vi "regressors.calculate.vi"(6 "reset? (F)":bool, 9 "initial_value (0)":dbl, 10 "variable v(k)":dbl, 11 "b0...bn":dbl[](array[numeric])=[0.0, 0.0, 0.0, 0.0]) -> (3 "result r(k)":dbl)   [LabVIEW 2015, in "discrete_control_systems.lvlib"]
doc: "Calculates a difference equation of the form r(k) = c0*v(k) + c1*v(k-1) + c2*v(k-2) .... cn*v(k-n) \n\nThe reset? input clears registers and intializes them to the specified initial value."
uses:
  discrete_control_systems.lvlib
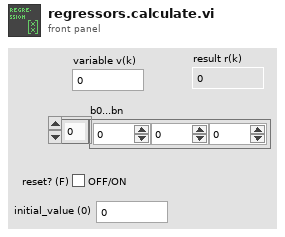
[diagram p1: front panel]
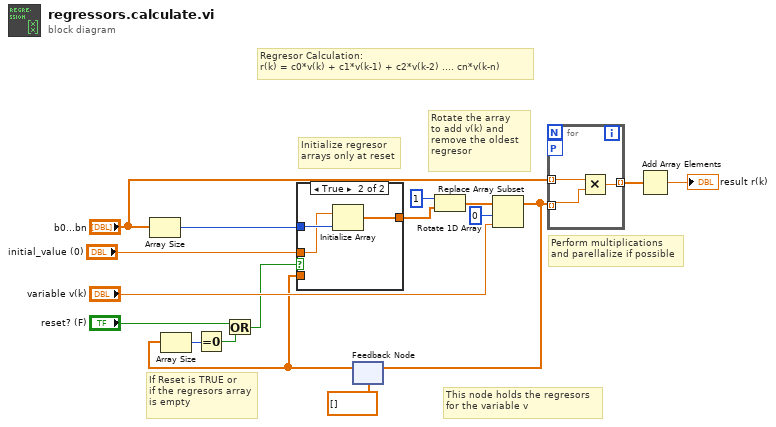
[diagram p0: block diagram]
diagram:
  # "If Reset is TRUE or\nif the regresors array\nis empty"
  # "Perform multiplications\nand parellalize if possible"
  # "Regresor Calculation:\nr(k) = c0*v(k) + c1*v(k-1) + c2*v(k-2) .... cn*v(k-n)"
  # "Initialize regresor\narrays only at reset"
  # "Rotate the array\nto add v(k) and \nremove the oldest \nregresor"
  # "This node holds the regresors\nfor the variable v"
  n1 = Array Size(array="b0...bn") -> (size(s)=w16:i32)
  n2 = feedback #1(dbl[] []) -> (w4:dbl[])
  n3 = Array Size(array=w4) -> (size(s)=w1:i32)
  n4 = Equal To 0?(x=w1) -> (x = 0?=w2:bool)
  n5 = Or(x="reset? (F)", y=w2) -> (x .or. y?=w5:bool)
  n6 = case shown="True" w5 {
    tunnel: w16 -> [_ w21]
    tunnel: [w18 w20] -> w14
    tunnel: w4 -> [w18 _]
    tunnel: "initial_value (0)" -> [_ w19]
    frame False {
    }
    frame True {
      n7 = Initialize Array(w19, w21) -> (w20:dbl[])
    }
  }
  n8 = Rotate 1D Array(1:w14, 2:1 ("n")) -> (0:w12:dbl[])
  n9 = Replace Array Subset(array=w12, new element="variable v(k)", index=0) -> (w6:dbl[])
  n10 = feedback-in #1(w6) -> ()
  n11 = for {
    tunnel: w6 -> [w24] mode=indexing
    tunnel: "b0...bn" -> [w23] mode=indexing
    tunnel: [w22] -> w9 mode=indexing
    workers-P: _ -> [_]
    n12 = Multiply(x=w23, y=w24) -> (x*y=w22:dbl)
  }
  n13 = Add Array Elements(numeric array=w9) -> (sum=→"result r(k)":dbl)
